vi "Autosize Listbox Columns.vi"(4 "error in (no error)":errorcluster, 6 "Resize Table?":bool, 7 "MCListbox Refnum":refnum<vi>) -> (0 "error out":errorcluster)   [LabVIEW 2014]
doc: "This VI resizes each column of the table specified by Table Ref based on the widest entry of the column. Additionally, if Resize Table? is TRUE, the VI will set the table width based on the number of populated columns."
panel:
  in  "Limit Rows to san to100? (T)":bool=TRUE
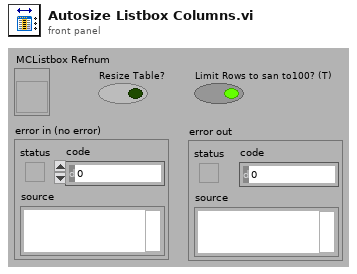
[diagram p1: front panel]
types:
  T1 = enum16{"User-specified Font", "Application Font", "System Font", "Dialog Font"}
  T2 = cluster{"Font Name:":string, "Size":i16, "Strikeout?":bool, "Italic?":bool, "Underline?":bool, "Outline?":bool, "Shadow?":bool, "Bold?":bool}
  T3 = cluster{"left":i16, "top":i16, "right":i16, "bottom":i16}
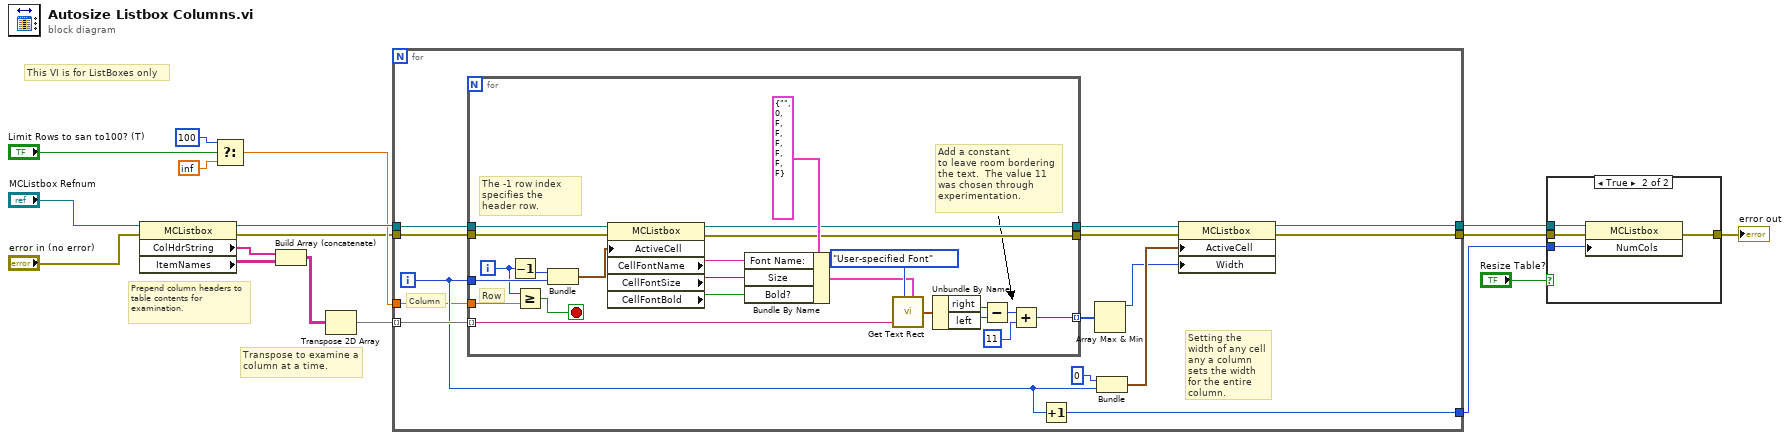
[diagram p0: block diagram]
diagram:
  # "This VI is for ListBoxes only"
  # "Transpose to examine a column at a time."
  # "Prepend column headers to table contents for examination."
  n1 = property class="MCListbox"(reference="MCListbox Refnum", error in="error in (no error)") -> (reference out=w17:refnum<vi>, error out=w1:errorcluster, "ColHdrString"=w16:string[], "ItemNames"=w13:string[][])
  n2 = Select(t=100 ("Timer ID (In)"), s="Limit Rows to san to100? (T)", f=inf) -> (s? t:f=w2:dbl)
  n3 = Build Array (concatenate)(w16, w13) -> (w15:string[][])
  n4 = Transpose 2D Array(2D array=w15) -> (transposed array=w14:string[][])
  n5 = for {
    tunnel: w14 -> [w31] mode=indexing
    tunnel: w17 -> [w18]
    tunnel: w1 -> [w19]
    tunnel: [w20] -> w9
    tunnel: [w24] -> w10
    tunnel: [w22] -> w8
    tunnel: w2 -> [w21]
    i -> [w23]
    # "Setting the width of any cell any a column sets the width for the entire column."
    # "Column"
    n6 = for {
      tunnel: w31 -> [w47] mode=indexing
      tunnel: w18 -> [w54]
      tunnel: w23 -> [w34]
      tunnel: [w37] -> w30 mode=indexing
      tunnel: w19 -> [w42]
      tunnel: [w41] -> w28
      tunnel: [w40] -> w29
      tunnel: w21 -> [w33]
      i -> [w32]
      stop <- w35 stop-if-true
      # "The -1 row index specifies the header row."
      # "Add a constant\nto leave room bordering the text.  The value 11 was chosen through experimentation."
      # "Row"
      n7 = Decrement(x=w32) -> (x-1=w43:i32)
      n8 = Greater Or Equal?(x=w32, y=w33) -> (x >= y?=w35:bool)
      n9 = Bundle(w43, w34) -> (w53:cluster{i32, i32})  [unwired: 1 in]
      n10 = property class="MCListbox"(reference=w54, error in=w42, "ActiveCell"=w53) -> (reference out=w40:refnum<vi>, error out=w41:errorcluster, "CellFontName"=w51:string, "CellFontSize"=w38:u32, "CellFontBold"=w50:bool)
      n11 = Bundle By Name(cluster=T2 {"Font Name:"="", "Size"=0, "Strikeout?"=FALSE, "Italic?"=FALSE, "Underline?"=FALSE, "Outline?"=FALSE, "Shadow?"=FALSE, "Bold?"=FALSE} ("[user-specified font]"), "Font Name:"=w51, "Size"=w38, "Bold?"=w50) -> (w48:T2)
      n12 = call <vilib>:"Get Text Rect.vi"("desired font(Application)"=T1."User-specified Font", "text"=w47, "[user-specified font]"=w48) -> ("rect"=w46:T3)  [unwired: 6 in]
      n13 = Unbundle By Name(w46) -> ("right"=w45:i16, "left"=w44:i16)
      n14 = Subtract(x=w45, y=w44) -> (x-y=w39:i16)
      n15 = Add(x=w39, y=i16 11) -> (x+y=w37:i16)
    }
    n16 = Increment(x=w23) -> (x+1=w22:i32)
    n17 = Array Max & Min(array=w30) -> (max value=w25:i16)  [unwired: 3 out]
    n18 = Bundle(0, w23) -> (w26:cluster{i32, i32})  [unwired: 1 in]
    n19 = property class="MCListbox"(reference=w29, error in=w28, "ActiveCell"=w26, "Width"=w25) -> (reference out=w24:refnum<vi>, error out=w20:errorcluster)
  }
  n20 = case shown="True" "Resize Table?" {
    tunnel: w10 -> [_ w59]
    tunnel: w9 -> [w55 w58]
    tunnel: w8 -> [_ w57]
    tunnel: [w55 w56] -> w7
    frame False {
    }
    frame True {
      n21 = property class="MCListbox"(reference=w59, error in=w58, "NumCols"=w57) -> (error out=w56:errorcluster)  [unwired: 1 out]
    }
  }
  "error out" <- w7
